vi "RichToFlatniswitch_grpc_GetRelayPositionResponse.vi"(5 "OutputClusterType":T1, 11 "InputCluster":T3) -> (3 "OutputCluster":T1)   [LabVIEW 2021, in "NI Switch_client.lvlib"]
uses:
  NI Switch_client.lvlib
  niswitch_grpc_RelayPosition.ctl
  niswitch_grpc_GetRelayPositionResponse_Flat.ctl
  niswitch_grpc_GetRelayPositionResponse.ctl
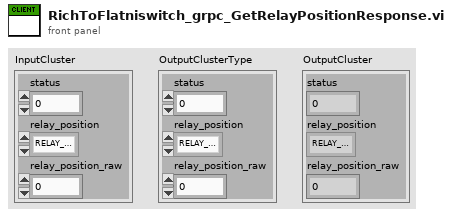
[diagram p1: front panel]
types:
  T1 = typedef "NI Switch_client.lvlib/niswitch_grpc_GetRelayPositionResponse_Flat.ctl" = cluster{"status":i32, "relay_position":T2, "relay_position_raw":i32}
  T2 = typedef "NI Switch_client.lvlib/niswitch_grpc_RelayPosition.ctl" = enum32{"RELAY_POSITION_UNSPECIFIED", "RELAY_POSITION_NISWITCH_VAL_OPEN", "RELAY_POSITION_NISWITCH_VAL_CLOSED"}
  T3 = typedef "NI Switch_client.lvlib/niswitch_grpc_GetRelayPositionResponse.ctl" = cluster{"status":i32, "relay_position":T2, "relay_position_raw":i32}
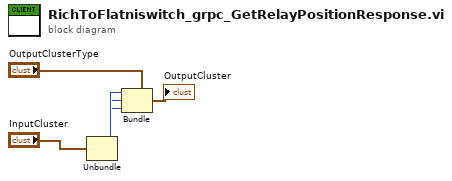
[diagram p0: block diagram]
diagram:
  n1 = Unbundle "Unbundle"("InputCluster") -> ("status"=w3:i32, "relay_position"=w2:T2, "relay_position_raw"=w1:i32)
  n2 = Bundle "Bundle"(cluster="OutputClusterType", "status"=w3, "relay_position"=w2, "relay_position_raw"=w1) -> (→"OutputCluster":T1)
